vi "SMTP Email GMT Delta.vi"() -> (0 "GMT Delta in seconds":dbl format="%0.2f")   [LabVIEW 2012, in "NewNI_SMTPEmail.lvlib"]
doc: "Returns this time zone's offset in seconds with respect to GMT."
uses:
  NewNI_SMTPEmail.lvlib
panel:
  in  "2 Jan 1980 00:00:00 GMT (in seconds)":dbl=2398464000.0 format="%0.2f"
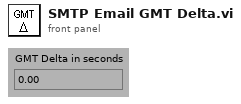
[diagram p1: front panel]
types:
  T1 = typedef "LVDateTimeRec.ctl" = cluster{"fractional second":dbl, "second":i32, "minute":i32, "hour":i32, "day of month":i32, "month":i32, "year":i32, "day of week":i32, "day of year":i32, "DST":i32}
  T2 = cluster{"second":i32, "minute":i32, "hour":i32, "day of month":i32, "month":i32, "year":i32, "day of week":i32, "day of year":i32, "is DST":i32}
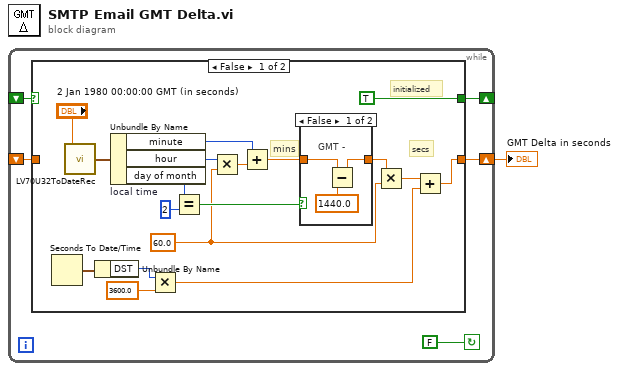
[diagram p0: block diagram]
diagram:
  n1 = while {
    shift-left: _ -> [w5]
    shift-right: [w4] -> _
    shift-left: _ -> [w3]
    shift-right: [w6] -> w1
    stop <- FALSE continue-if-true
    n2 = case shown="False" w5 {
      selector: w5 -> [_ w30]
      tunnel: [w7 w29] -> w6
      tunnel: [TRUE w30] -> w4
      tunnel: w3 -> [_ w29]
      frame False {
        w12 = 60.0
        # "initialized"
        # "mins"
        # "secs"
        n3 = Seconds To Date/Time() -> (date time rec=w13:T1)  [unwired: 2 out]
        n4 = call <vilib>:"LV70U32ToDateRec.vi"("Time"="2 Jan 1980 00:00:00 GMT (in seconds)") -> ("date time rec"=w24:T2)
        n5 = Unbundle By Name(w13) -> ("DST"=w11:i32)
        n6 = Unbundle By Name "local time"(w24) -> ("minute"=w15:i32, "hour"=w17:i32, "day of month"=w23:i32)
        n7 = Multiply(x=w11, y=3600.0) -> (x*y=w9:dbl)
        n8 = Equal?(x=w23, y=2) -> (x = y?=w21:bool)
        n9 = Multiply(x=w17, y=w12) -> (x*y=w16:dbl)
        n10 = Add(x=w15, y=w16) -> (x+y=w14:dbl)
        n11 = case shown="False" w21 {
          tunnel: [w27 w28] -> w18
          tunnel: w14 -> [w25 w28]
          frame False {
            # "GMT -"
            n12 = Subtract(x=w25, y=1440.0) -> (x-y=w27:dbl)
          }
          frame True {
            # "GMT +"
          }
        }
        n13 = Multiply(x=w18, y=w12) -> (x*y=w8:dbl)
        n14 = Add(x=w8, y=w9) -> (x+y=w7:dbl)
      }
      frame True {
        # "already initialized"
      }
    }
  }
  "GMT Delta in seconds" <- w1
